vi "client.vi"() -> ()   [LabVIEW 2015]
uses:
  Control/Queue.ctl
panel:
  in  "Operation":bool
  in  "Channel":enum16{"64X4", "128X4"}(ring)=enum."128X4"
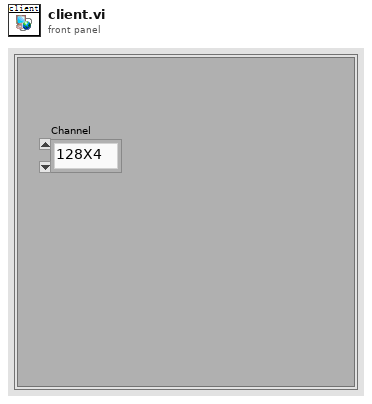
[diagram p1: front panel]
types:
  T1 = typedef "Queue.ctl" = cluster{"Panel":enum16{"None", "Password", "User", "Control", "Monitor", "Operation"}}
  T2 = enum16{"None", "Password", "User", "Control", "Monitor", "Operation"}
  T3 = enum32{"Bad", "Idle", "Run top level", "Running"}
  T4 = typedef "LVRectTypeDef.ctl" = cluster{"Left":i16, "Top":i16, "Right":i16, "Bottom":i16}
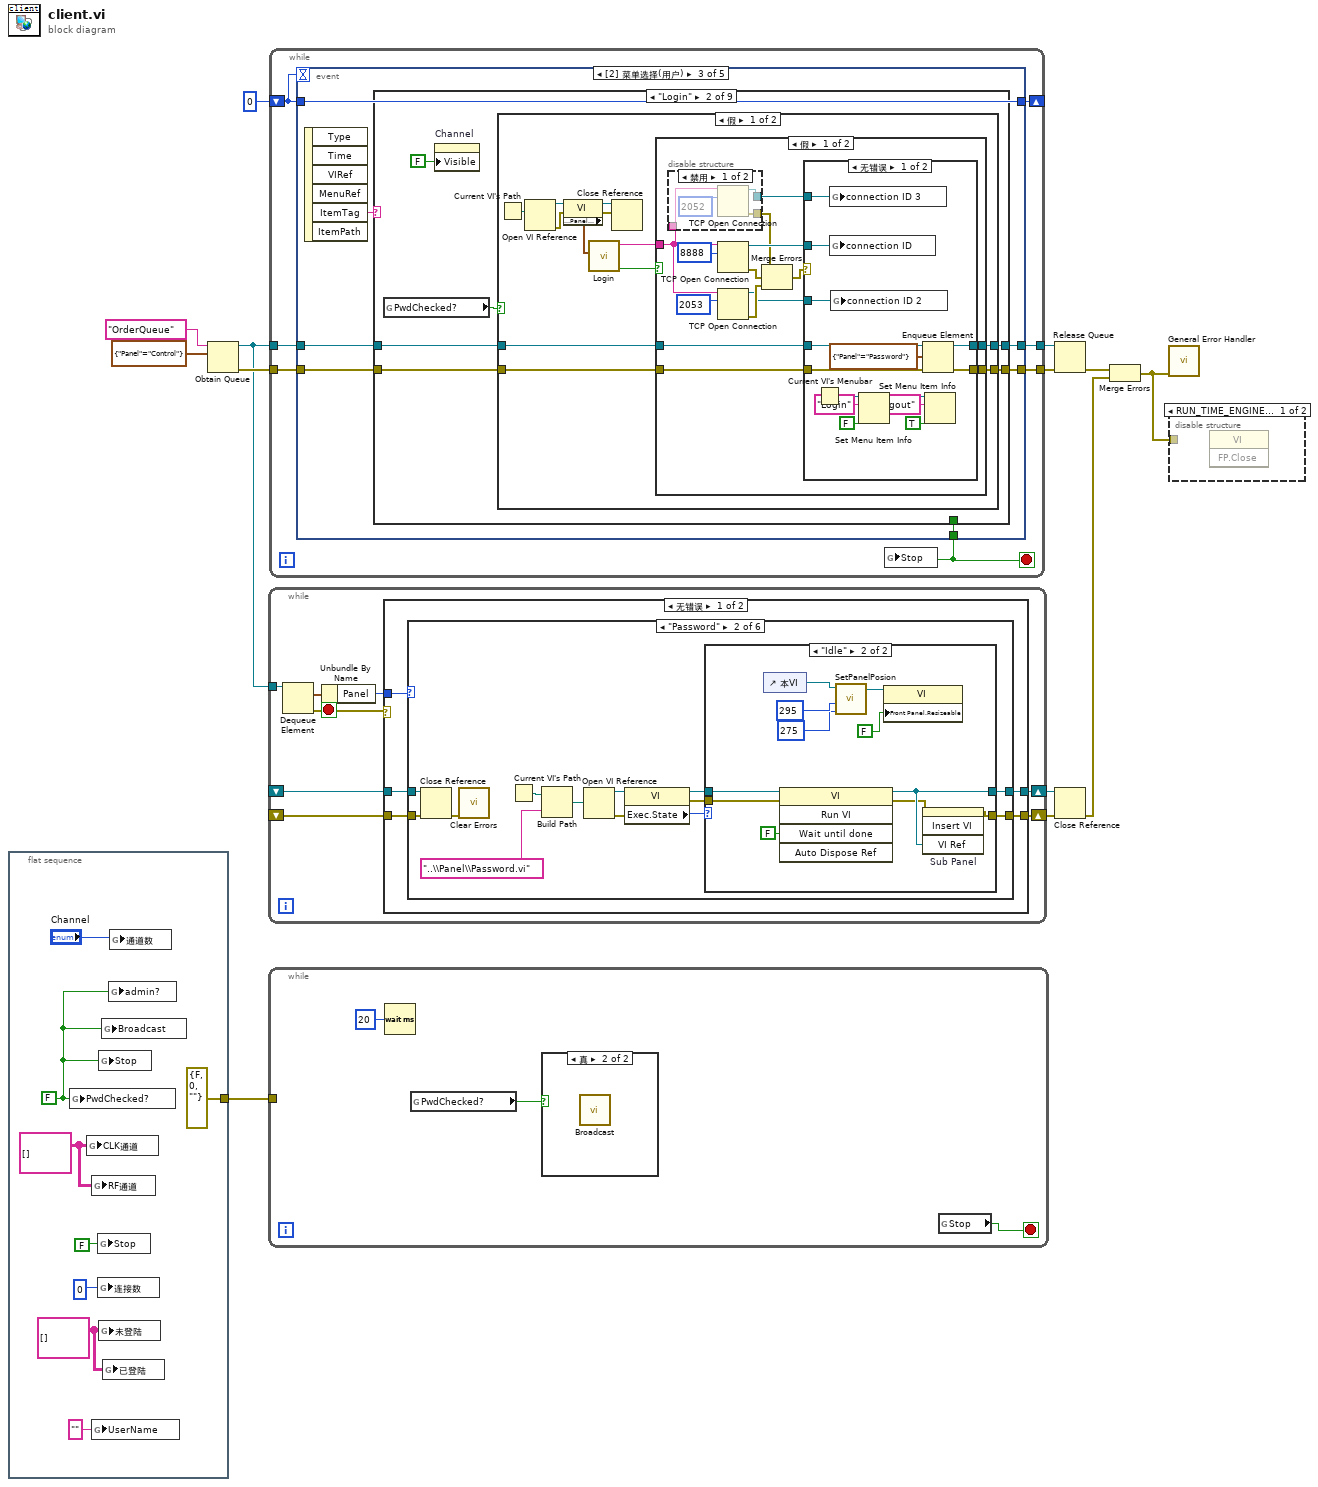
[diagram p0: block diagram]
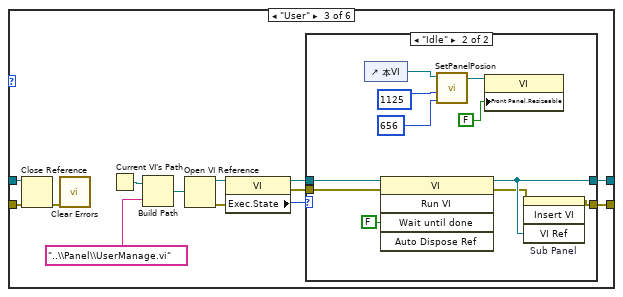
[diagram p6: hidden frame]
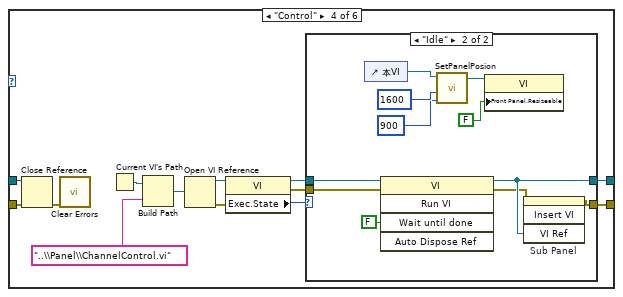
[diagram p8: hidden frame]
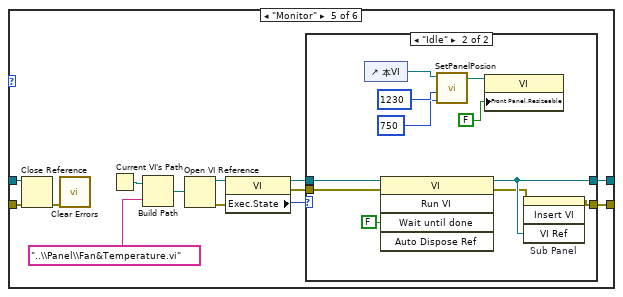
[diagram p10: hidden frame]
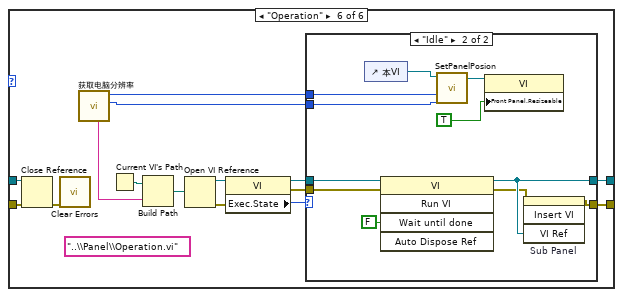
[diagram p12: hidden frame]
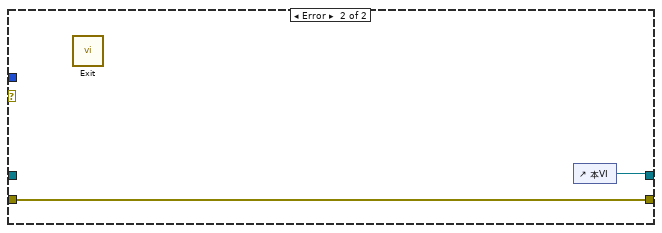
[diagram p14: hidden frame]
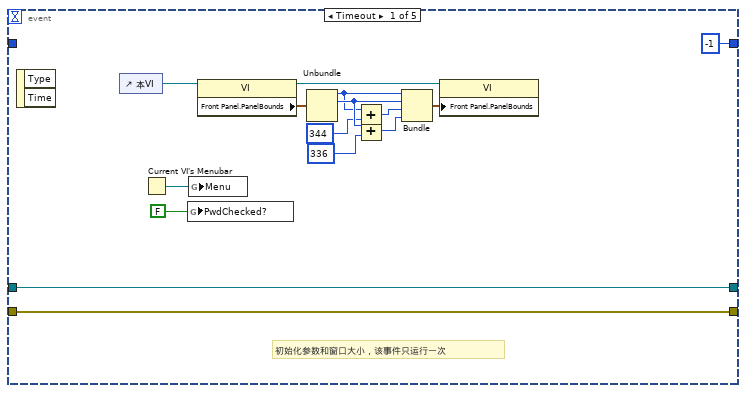
[diagram p15: hidden frame]
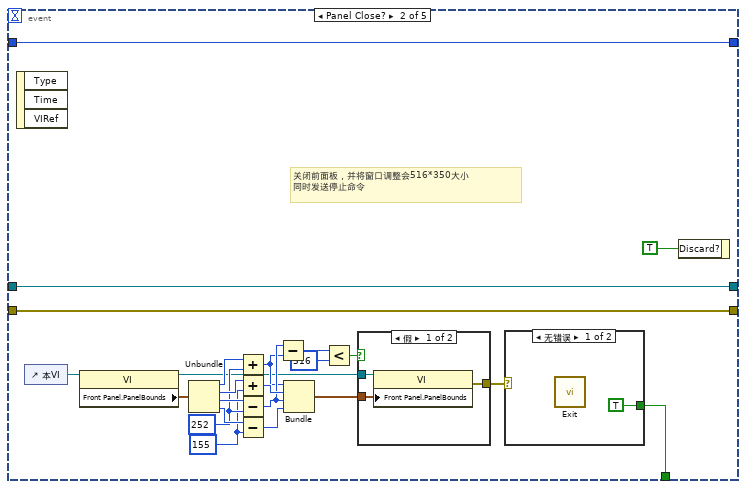
[diagram p16: hidden frame]
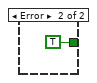
[diagram p18: hidden frame]
diagram:
  n1 = flat-sequence {
    tunnel: [errorcluster {"status"=FALSE, "code"=0, "source"=""} ("error constant")] -> w2
    frame #0 {
      w17 = string[][] [] ("未登陆")
      w20 = string[][] [] ("CLK通道")
      w16 = FALSE ("PwdChecked?")
      n2 = global write "Globalclient.vi" "PwdChecked?"(w16) -> ()
      n3 = global write "Globalclient.vi" "CLK通道"(w20) -> ()
      n4 = global write "Globalclient.vi" "RF通道"(w20) -> ()
      n5 = global write "Globalclient.vi" "UserName"("" ("UserName")) -> ()
      n6 = global write "Globalclient.vi" "Stop"(FALSE ("Stop")) -> ()
      n7 = global write "Globalclient.vi" "连接数"(0 ("连接数")) -> ()
      n8 = global write "Globalclient.vi" "Stop"(w16) -> ()
      n9 = global write "Globalclient.vi" "未登陆"(w17) -> ()
      n10 = global write "Globalclient.vi" "Broadcast"(w16) -> ()
      n11 = global write "Globalclient.vi" "已登陆"(w17) -> ()
      n12 = global write "Globalclient.vi" "admin?"(w16) -> ()
      n13 = global write "Globalclient.vi" "通道数"("Channel") -> ()
    }
  }
  n14 = Obtain Queue(name (unnamed)="OrderQueue" ("名称（未命名）"), element data type=T1 {"Panel"=enum."Control"}) -> (queue out=w8:refnum<queue>, error out=w11:errorcluster)  [unwired: 3 in, 1 out]
  n15 = while {
    tunnel: w8 -> [w29]
    shift-right: [w26] -> w7
    shift-left: _ -> [w24]
    shift-right: [w25] -> w6
    shift-left: _ -> [w23]
    stop <- w22 stop-if-true
    n16 = Dequeue Element(queue=w29) -> (element=w28:T1, error out=w22:errorcluster)  [unwired: 2 in, 2 out]
    n17 = Unbundle By Name(w28) -> ("Panel"=w27:T2)
    n18 = case shown="无错误" w22 {
      tunnel: w27 -> [w30 _]
      tunnel: [w34 w168] -> w26
      tunnel: [w33 w169] -> w25
      tunnel: w24 -> [w32 _]
      tunnel: w23 -> [w31 w169]
      frame No Error {
        n19 = case shown="\"Password\"" w30 {
          tunnel: [_ w47 w73 w99 w125 w154] -> w34
          tunnel: [w35 w45 w71 w97 w123 w152] -> w33
          tunnel: w32 -> [_ w44 w70 w96 w122 w151]
          tunnel: w31 -> [w35 w43 w69 w95 w121 w150]
          frame "None", Default {
          }
          frame "Password" {
            n20 = Close Reference(reference=w44, error in (no error)=w43) -> (error out=w46:errorcluster)
            n21 = call <vilib>:"Clear Errors.vi"("error in (no error)"=w46) -> ()  [unwired: 5 in, 2 out]
            n22 = Current VI's Path() -> (path=w37:path)
            n23 = Build Path(base path=w37, name or relative path="..\\Panel\\Password.vi" ("名称或相对路径")) -> (appended path=w36:path)
            n24 = Open VI Reference(vi path=w36) -> (vi reference=w42:refnum<vi>, error out=w40:errorcluster)  [unwired: 5 in]
            n25 = property class="VI"(reference=w42, error in=w40) -> (reference out=w41:refnum<vi>, error out=w39:errorcluster, "Exec.State"=w38:T3)
            n26 = case shown="\"Idle\"" w38 {
              tunnel: [w49 w60] -> w47
              tunnel: [w50 w59] -> w45
              tunnel: w41 -> [w49 w57]
              tunnel: w39 -> [w50 w56]
              frame "Bad", Default {
              }
              frame "Idle" {
                n27 = control-ref of="本VI"() -> (w55:refnum<vi>)
                n28 = invoke class="VI" method="Run VI"(reference=w57, error in=w56, "Wait until done"=FALSE ("结束前等待")) -> (reference out=w60:refnum<vi>, error out=w58:errorcluster)  [unwired: 2 in, 3 out]
                n29 = call "SetPanelPosion.vi"("Bottom"=i16 275, "Right"=i16 295, "VI ref in"=w55) -> ("VI ref out"=w52:refnum<vi>)  [unwired: 8 in]
                n30 = property class="VI"(reference=w52, "Front Panel.Resizeable"=FALSE ("Front Panel Window:Resizable")) -> ()  [unwired: 1 in, 2 out]
                n31 = invoke on="Sub Panel" class="SubPnl" method="Insert VI"(error in=w58, "VI Ref"=w60) -> (error out=w59:errorcluster)  [unwired: 2 in, 3 out]
              }
            }
          }
          frame "User" {
            n32 = Close Reference(reference=w70, error in (no error)=w69) -> (error out=w72:errorcluster)
            n33 = call <vilib>:"Clear Errors.vi"("error in (no error)"=w72) -> ()  [unwired: 5 in, 2 out]
            n34 = Current VI's Path() -> (path=w63:path)
            n35 = Build Path(base path=w63, name or relative path="..\\Panel\\UserManage.vi" ("名称或相对路径")) -> (appended path=w62:path)
            n36 = Open VI Reference(vi path=w62) -> (vi reference=w68:refnum<vi>, error out=w66:errorcluster)  [unwired: 5 in]
            n37 = property class="VI"(reference=w68, error in=w66) -> (reference out=w67:refnum<vi>, error out=w65:errorcluster, "Exec.State"=w64:T3)
            n38 = case shown="\"Idle\"" w64 {
              tunnel: [w75 w86] -> w73
              tunnel: [w76 w85] -> w71
              tunnel: w67 -> [w75 w83]
              tunnel: w65 -> [w76 w82]
              frame "Bad", Default {
              }
              frame "Idle" {
                n39 = control-ref of="本VI"() -> (w81:refnum<vi>)
                n40 = invoke class="VI" method="Run VI"(reference=w83, error in=w82, "Wait until done"=FALSE ("结束前等待")) -> (reference out=w86:refnum<vi>, error out=w84:errorcluster)  [unwired: 2 in, 3 out]
                n41 = call "SetPanelPosion.vi"("Bottom"=i16 656, "Right"=i16 1125, "VI ref in"=w81) -> ("VI ref out"=w78:refnum<vi>)  [unwired: 8 in]
                n42 = property class="VI"(reference=w78, "Front Panel.Resizeable"=FALSE ("Front Panel Window:Resizable")) -> ()  [unwired: 1 in, 2 out]
                n43 = invoke on="Sub Panel" class="SubPnl" method="Insert VI"(error in=w84, "VI Ref"=w86) -> (error out=w85:errorcluster)  [unwired: 2 in, 3 out]
              }
            }
          }
          frame "Control" {
            n44 = Close Reference(reference=w96, error in (no error)=w95) -> (error out=w98:errorcluster)
            n45 = call <vilib>:"Clear Errors.vi"("error in (no error)"=w98) -> ()  [unwired: 5 in, 2 out]
            n46 = Current VI's Path() -> (path=w89:path)
            n47 = Build Path(base path=w89, name or relative path="..\\Panel\\ChannelControl.vi" ("名称或相对路径")) -> (appended path=w88:path)
            n48 = Open VI Reference(vi path=w88) -> (vi reference=w94:refnum<vi>, error out=w92:errorcluster)  [unwired: 5 in]
            n49 = property class="VI"(reference=w94, error in=w92) -> (reference out=w93:refnum<vi>, error out=w91:errorcluster, "Exec.State"=w90:T3)
            n50 = case shown="\"Idle\"" w90 {
              tunnel: [w101 w112] -> w99
              tunnel: [w102 w111] -> w97
              tunnel: w93 -> [w101 w109]
              tunnel: w91 -> [w102 w108]
              frame "Bad", Default {
              }
              frame "Idle" {
                n51 = control-ref of="本VI"() -> (w107:refnum<vi>)
                n52 = invoke class="VI" method="Run VI"(reference=w109, error in=w108, "Wait until done"=FALSE ("结束前等待")) -> (reference out=w112:refnum<vi>, error out=w110:errorcluster)  [unwired: 2 in, 3 out]
                n53 = call "SetPanelPosion.vi"("Bottom"=i16 900, "Right"=i16 1600, "VI ref in"=w107) -> ("VI ref out"=w104:refnum<vi>)  [unwired: 8 in]
                n54 = property class="VI"(reference=w104, "Front Panel.Resizeable"=FALSE ("Front Panel Window:Resizable")) -> ()  [unwired: 1 in, 2 out]
                n55 = invoke on="Sub Panel" class="SubPnl" method="Insert VI"(error in=w110, "VI Ref"=w112) -> (error out=w111:errorcluster)  [unwired: 2 in, 3 out]
              }
            }
          }
          frame "Monitor" {
            n56 = Close Reference(reference=w122, error in (no error)=w121) -> (error out=w124:errorcluster)
            n57 = call <vilib>:"Clear Errors.vi"("error in (no error)"=w124) -> ()  [unwired: 5 in, 2 out]
            n58 = Current VI's Path() -> (path=w115:path)
            n59 = Build Path(base path=w115, name or relative path="..\\Panel\\Fan&Temperature.vi" ("名称或相对路径")) -> (appended path=w114:path)
            n60 = Open VI Reference(vi path=w114) -> (vi reference=w120:refnum<vi>, error out=w118:errorcluster)  [unwired: 5 in]
            n61 = property class="VI"(reference=w120, error in=w118) -> (reference out=w119:refnum<vi>, error out=w117:errorcluster, "Exec.State"=w116:T3)
            n62 = case shown="\"Idle\"" w116 {
              tunnel: [w127 w138] -> w125
              tunnel: [w128 w137] -> w123
              tunnel: w119 -> [w127 w135]
              tunnel: w117 -> [w128 w134]
              frame "Bad", Default {
              }
              frame "Idle" {
                n63 = control-ref of="本VI"() -> (w133:refnum<vi>)
                n64 = invoke class="VI" method="Run VI"(reference=w135, error in=w134, "Wait until done"=FALSE ("结束前等待")) -> (reference out=w138:refnum<vi>, error out=w136:errorcluster)  [unwired: 2 in, 3 out]
                n65 = call "SetPanelPosion.vi"("Bottom"=i16 750, "Right"=i16 1230, "VI ref in"=w133) -> ("VI ref out"=w130:refnum<vi>)  [unwired: 8 in]
                n66 = property class="VI"(reference=w130, "Front Panel.Resizeable"=FALSE ("Front Panel Window:Resizable")) -> ()  [unwired: 1 in, 2 out]
                n67 = invoke on="Sub Panel" class="SubPnl" method="Insert VI"(error in=w136, "VI Ref"=w138) -> (error out=w137:errorcluster)  [unwired: 2 in, 3 out]
              }
            }
          }
          frame "Operation" {
            (unwired) "..\\Panel\\Operation.vi" ("名称或相对路径")
            n68 = Close Reference(reference=w151, error in (no error)=w150) -> (error out=w153:errorcluster)
            n69 = call <vilib>:"Clear Errors.vi"("error in (no error)"=w153) -> ()  [unwired: 5 in, 2 out]
            n70 = call "获取电脑分辨率.vi"() -> ("宽"=w140:i32, "长"=w141:i32, "子面板路径"=w142:string)  [unwired: 9 in]
            n71 = Current VI's Path() -> (path=w144:path)
            n72 = Build Path(base path=w144, name or relative path=w142) -> (appended path=w143:path)
            n73 = Open VI Reference(vi path=w143) -> (vi reference=w149:refnum<vi>, error out=w147:errorcluster)  [unwired: 5 in]
            n74 = property class="VI"(reference=w149, error in=w147) -> (reference out=w148:refnum<vi>, error out=w146:errorcluster, "Exec.State"=w145:T3)
            n75 = case shown="\"Idle\"" w145 {
              tunnel: [w155 w166] -> w154
              tunnel: [w156 w165] -> w152
              tunnel: w148 -> [w155 w163]
              tunnel: w146 -> [w156 w162]
              tunnel: w141 -> [_ w158]
              tunnel: w140 -> [_ w157]
              frame "Bad", Default {
              }
              frame "Idle" {
                n76 = control-ref of="本VI"() -> (w161:refnum<vi>)
                n77 = invoke class="VI" method="Run VI"(reference=w163, error in=w162, "Wait until done"=FALSE ("结束前等待")) -> (reference out=w166:refnum<vi>, error out=w164:errorcluster)  [unwired: 2 in, 3 out]
                n78 = call "SetPanelPosion.vi"("Bottom"=w157, "Right"=w158, "VI ref in"=w161) -> ("VI ref out"=w160:refnum<vi>)  [unwired: 8 in]
                n79 = property class="VI"(reference=w160, "Front Panel.Resizeable"=TRUE ("Front Panel Window:Resizable")) -> ()  [unwired: 1 in, 2 out]
                n80 = invoke on="Sub Panel" class="SubPnl" method="Insert VI"(error in=w164, "VI Ref"=w166) -> (error out=w165:errorcluster)  [unwired: 2 in, 3 out]
              }
            }
          }
        }
      }
      frame Error {
        n81 = call "Exit.vi"() -> ()  [unwired: 12 in]
        n82 = control-ref of="本VI"() -> (w168:refnum<vi>)
      }
    }
  }
  n83 = while {
    tunnel: w2 -> [_]
    stop <- w170 stop-if-true
    n84 = Wait (ms)(milliseconds to wait=u32 20) -> ()  [unwired: 1 out]
    n85 = global read "Globalclient.vi" "PwdChecked?"() -> (w172:bool)
    n86 = case shown="真" w172 {
      frame False {
      }
      frame True {
        n87 = call "Broadcast.vi"() -> ()  [unwired: 20 in]
      }
    }
    n88 = global read "Globalclient.vi" "Stop"() -> (w170:bool)
  }
  n89 = while {
    tunnel: w8 -> [w179]
    tunnel: [w178] -> w10
    tunnel: w11 -> [w177]
    tunnel: [w176] -> w9
    shift-right: [w175] -> _
    shift-left: 0 -> [w174]
    stop <- w173 stop-if-true
    n90 = event shown="[2] 菜单选择(用户)" {
      selector: _ -> [_ _ _ _ _]
      dyn-events: _ -> [_ _ _ _ _]
      timeout: w174 -> [_ _ _ _ _]
      tunnel: [_ w214 w228 _ _] -> w173
      tunnel: w179 -> [w193 w216 w227 w393 w399]
      tunnel: [w194 w217 w226 w394 w396] -> w178
      tunnel: w177 -> [w194 w217 w225 w394 w397]
      tunnel: [w193 w216 w224 w393 w398] -> w176
      tunnel: [-1 w213 w223 _ _] -> w175
      tunnel: w174 -> [_ w213 w223 _ _]
      event Timeout {
        # "初始化参数和窗口大小，该事件只运行一次"
        n91 = event-data() -> ()  [unwired: 1 in, 2 out]
        n92 = control-ref of="本VI"() -> (w192:refnum<vi>)
        n93 = Current VI's Menubar() -> (w181:refnum<k9>)
        n94 = global write "Globalclient.vi" "PwdChecked?"(FALSE ("PwdChecked?")) -> ()
        n95 = global write "Globalclient.vi" "Menu"(w181) -> ()
        n96 = property class="VI"(reference=w192) -> (reference out=w183:refnum<vi>, "Front Panel.PanelBounds"=w184:T4)  [unwired: 1 in, 1 out]
        n97 = Unbundle(w184) -> ("Left"=w187:i16, "Top"=w188:i16)  [unwired: 2 out]
        n98 = Add(x=w187, y=i16 344 ("Right")) -> (x+y=w189:i16)
        n99 = Add(x=w188, y=i16 336 ("Bottom")) -> (x+y=w190:i16)
        n100 = Bundle("Left"=w187, "Top"=w188, w189, w190) -> (w191:cluster{"Left":i16, "Top":i16, i16, i16})  [unwired: 1 in]
        n101 = property class="VI"(reference=w183, "Front Panel.PanelBounds"=w191) -> ()  [unwired: 1 in, 2 out]
      }
      event Panel Close? {
        w202 = i16 155 ("Bottom")
        w203 = i16 252 ("Right")
        # "关闭前面板，并将窗口调整会516*350大小\n同时发送停止命令"
        n102 = event-data() -> ()  [unwired: 1 in, 3 out]
        n103 = control-ref of="本VI"() -> (w211:refnum<vi>)
        n104 = property class="VI"(reference=w211) -> (reference out=w197:refnum<vi>, "Front Panel.PanelBounds"=w208:T4)  [unwired: 1 in, 1 out]
        n105 = Unbundle(w208) -> ("Left"=w209:i16, "Top"=w206:i16, "Right"=w205:i16, "Bottom"=w204:i16)
        n106 = Add(x=w209, y=w203) -> (x+y=w199:i16)
        n107 = Add(x=w206, y=w202) -> (x+y=w207:i16)
        n108 = Subtract(x=w205, y=w203) -> (x-y=w200:i16)
        n109 = Subtract(x=w204, y=w202) -> (x-y=w210:i16)
        n110 = Subtract(x=w200, y=w199) -> (x-y=w201:i16)
        n111 = Bundle(w199, w207, w200, w210) -> (w196:cluster{i16, i16, i16, i16})  [unwired: 1 in]
        n112 = Less?(x=w201, y=i16 516) -> (x < y?=w195:bool)
        n113 = case shown="假" w195 {
          tunnel: w197 -> [w220 _]
          tunnel: w196 -> [w219 _]
          tunnel: [w218 _] -> w212
          frame False {
            n114 = property class="VI"(reference=w220, "Front Panel.PanelBounds"=w219) -> (error out=w218:errorcluster)  [unwired: 1 in, 1 out]
          }
          frame True {
          }
        }
        n115 = case shown="无错误" w212 {
          tunnel: [TRUE TRUE] -> w214
          frame No Error {
            n116 = call "Exit.vi"() -> ()  [unwired: 12 in]
          }
          frame Error {
          }
        }
        n117 = event-data("Discard?"=TRUE ("放弃？")) -> ()  [unwired: 1 in, 1 out]
      }
      event Menu Selection (User) {
        n118 = event-data() -> ("ItemTag"=w229:string)  [unwired: 1 in, 5 out]
        n119 = case shown="\"Login\"" w229 {
          tunnel: [_ _ _ _ _ _ _ w376 _] -> w228
          tunnel: w227 -> [w231 w237 w293 w335 w340 w345 w349 w378 w390]
          tunnel: [w230 w236 w291 w332 w337 w342 w346 w377 w391] -> w226
          tunnel: w225 -> [w230 w235 w292 w333 w338 w343 w347 w377 w391]
          tunnel: [w231 w234 w290 w334 w339 w344 w348 w378 w390] -> w224
          frame "假", Default {
          }
          frame "Login" {
            n120 = global read "Globalclient.vi" "PwdChecked?"() -> (w233:bool)
            n121 = property on="Channel" class="Enum (严格)"("Visible"=FALSE ("可见")) -> ()  [unwired: 2 in, 2 out]
            n122 = case shown="假" w233 {
              tunnel: w237 -> [w244 w289]
              tunnel: [w243 w288] -> w236
              tunnel: w235 -> [w242 w288]
              tunnel: [w241 w289] -> w234
              frame False {
                n123 = Current VI's Path() -> (path=w249:path)
                n124 = Open VI Reference(vi path=w249) -> (vi reference=w248:refnum<vi>, error out=w247:errorcluster)  [unwired: 5 in]
                n125 = property class="VI"(reference=w248, error in=w247) -> (reference out=w245:refnum<vi>, error out=w246:errorcluster, "Front Panel.PanelBounds"=w240:T4)
                n126 = call "Login.vi"("窗口边界"=w240) -> ("drop?"=w238:bool, "User IP"=w239:string)  [unwired: 9 in]
                n127 = Close Reference(reference=w245, error in (no error)=w246) -> ()  [unwired: 1 out]
                n128 = case shown="假" w238 {
                  tunnel: w239 -> [w252 _]
                  tunnel: w244 -> [w261 w286]
                  tunnel: [w260 w285] -> w243
                  tunnel: w242 -> [w259 w285]
                  tunnel: [w258 w286] -> w241
                  frame False {
                    n129 = disable-structure shown="禁用" {
                      disable-tunnel: [w266 _] -> w253
                      disable-tunnel: w252 -> [w265 _]
                      disable-tunnel: [w264 _] -> w251
                      frame Disabled {
                        n130 = TCP Open Connection(address=w265, remote port or service name=u32 2052 ("远程端口或服务名称")) -> (connection ID=w266:refnum<k5>, error out=w264:errorcluster)  [unwired: 3 in]
                      }
                      frame Enabled {
                      }
                    }
                    n131 = TCP Open Connection(address=w252, remote port or service name=u32 8888 ("远程端口或服务名称")) -> (connection ID=w262:refnum<k5>, error out=w257:errorcluster)  [unwired: 3 in]
                    n132 = TCP Open Connection(address=w252, remote port or service name=u32 2053 ("远程端口或服务名称")) -> (connection ID=w254:refnum<k5>, error out=w256:errorcluster)  [unwired: 3 in]
                    n133 = Merge Errors(w251, w257, w256) -> (w255:errorcluster)
                    n134 = case shown="无错误" w255 {
                      tunnel: w262 -> [w271 _]
                      tunnel: w261 -> [w281 w284]
                      tunnel: [w279 w283] -> w260
                      tunnel: w259 -> [w280 w283]
                      tunnel: [w278 w284] -> w258
                      tunnel: w254 -> [w269 _]
                      tunnel: w253 -> [w268 _]
                      frame No Error {
                        n135 = Current VI's Menubar() -> (w277:refnum<k9>)
                        n136 = global write "Globalclient.vi" "connection ID 3"(w268) -> ()
                        n137 = global write "Globalclient.vi" "connection ID"(w271) -> ()
                        n138 = global write "Globalclient.vi" "connection ID 2"(w269) -> ()
                        n139 = Set Menu Item Info(7:"Login" ("项名称"), 9:FALSE ("已启用"), 11:w277) -> (3:w276:refnum<k9>)  [unwired: 4 in, 1 out]
                        n140 = Enqueue Element(queue=w281, element=T1 {"Panel"=enum."Password"}, error in (no error)=w280) -> (queue out=w278:refnum<queue>, error out=w279:errorcluster)  [unwired: 1 in, 1 out]
                        n141 = Set Menu Item Info(7:"Logout" ("项名称"), 9:TRUE ("已启用"), 11:w276) -> ()  [unwired: 4 in, 2 out]
                      }
                      frame Error {
                        n142 = One Button Dialog(message="Link failure!" ("消息")) -> ()  [unwired: 1 in, 1 out]
                      }
                    }
                  }
                  frame True {
                  }
                }
              }
              frame True {
                n143 = One Button Dialog(message="Server connected!" ("消息")) -> ()  [unwired: 1 in, 1 out]
              }
            }
          }
          frame "Logout" {
            w300 = i16 155 ("Bottom")
            w301 = i16 252 ("Right")
            n144 = control-ref of="本VI"() -> (w311:refnum<vi>)
            n145 = property class="VI"(reference=w311) -> (reference out=w307:refnum<vi>, "Front Panel.PanelBounds"=w308:T4)  [unwired: 1 in, 1 out]
            n146 = Unbundle(w308) -> ("Left"=w309:i16, "Top"=w304:i16, "Right"=w303:i16, "Bottom"=w302:i16)
            n147 = Add(x=w309, y=w301) -> (x+y=w295:i16)
            n148 = Add(x=w304, y=w300) -> (x+y=w305:i16)
            n149 = Subtract(x=w303, y=w301) -> (x-y=w296:i16)
            n150 = Subtract(x=w302, y=w300) -> (x-y=w310:i16)
            n151 = Subtract(x=w296, y=w295) -> (x-y=w297:i16)
            n152 = Bundle(w295, w305, w296, w310) -> (w306:cluster{i16, i16, i16, i16})  [unwired: 1 in]
            n153 = Less?(x=w297, y=i16 516) -> (x < y?=w299:bool)
            n154 = case shown="真" w299 {
              tunnel: w307 -> [w314 _]
              tunnel: w306 -> [w313 _]
              tunnel: [w312 _] -> w298
              frame False {
                n155 = property class="VI"(reference=w314, "Front Panel.PanelBounds"=w313) -> (error out=w312:errorcluster)  [unwired: 1 in, 1 out]
              }
              frame True {
              }
            }
            n156 = case shown="无错误" w298 {
              tunnel: w293 -> [w318 w330]
              tunnel: w292 -> [w317 w329]
              tunnel: [w317 w329] -> w291
              tunnel: [w318 w330] -> w290
              frame No Error {
                n157 = global write "Globalclient.vi" "PwdChecked?"(FALSE ("PwdChecked?")) -> ()
                n158 = invoke on="Sub Panel" class="SubPanel" method="Remove VI"() -> ()  [unwired: 3 in, 3 out]
                n159 = Current VI's Menubar() -> (w327:refnum<k9>)
                n160 = call "Exit.vi"() -> ()  [unwired: 12 in]
                n161 = Set Menu Item Info(7:"Login" ("项名称"), 9:TRUE ("已启用"), 11:w327) -> (0:w322:errorcluster, 3:w326:refnum<k9>)  [unwired: 4 in]
                n162 = Set Menu Item Info(7:"Logout" ("项名称"), 8:w322, 9:FALSE ("已启用"), 11:w326) -> (0:w321:errorcluster, 3:w323:refnum<k9>)  [unwired: 3 in]
                n163 = Delete Menu Items(6:w321, 7:"Operation" ("项"), 9:w323) -> (0:w315:errorcluster)  [unwired: 1 in, 1 out]
                n164 = call <vilib>:"Clear Errors.vi"("error in (no error)"=w315) -> ()  [unwired: 5 in, 2 out]
              }
              frame Error {
              }
            }
          }
          frame "User" {
            n165 = Enqueue Element(queue=w335, element=T1 {"Panel"=enum."User"}, error in (no error)=w333) -> (queue out=w334:refnum<queue>, error out=w332:errorcluster)  [unwired: 1 in, 1 out]
          }
          frame "Control" {
            n166 = Enqueue Element(queue=w340, element=T1 {"Panel"=enum."Control"}, error in (no error)=w338) -> (queue out=w339:refnum<queue>, error out=w337:errorcluster)  [unwired: 1 in, 1 out]
          }
          frame "Monitor" {
            n167 = Enqueue Element(queue=w345, element=T1 {"Panel"=enum."Monitor"}, error in (no error)=w343) -> (queue out=w344:refnum<queue>, error out=w342:errorcluster)  [unwired: 1 in, 1 out]
          }
          frame "Operation" {
            n168 = disable-structure shown="Enabled" {
              disable-tunnel: w349 -> [w353 w356]
              disable-tunnel: [w352 w356] -> w348
              disable-tunnel: w347 -> [w351 w355]
              disable-tunnel: [w350 w355] -> w346
              frame Enabled {
                n169 = Enqueue Element(queue=w353, element=T1 {"Panel"=enum."Operation"}, error in (no error)=w351) -> (queue out=w352:refnum<queue>, error out=w350:errorcluster)  [unwired: 1 in, 1 out]
              }
              frame Disabled {
              }
            }
          }
          frame "Exit" {
            w364 = i16 155 ("Bottom")
            w365 = i16 252 ("Right")
            n170 = control-ref of="本VI"() -> (w375:refnum<vi>)
            n171 = property class="VI"(reference=w375) -> (reference out=w371:refnum<vi>, "Front Panel.PanelBounds"=w372:T4)  [unwired: 1 in, 1 out]
            n172 = property on="Channel" class="Enum (严格)"("Visible"=TRUE ("可见")) -> ()  [unwired: 2 in, 2 out]
            n173 = Unbundle(w372) -> ("Left"=w373:i16, "Top"=w368:i16, "Right"=w367:i16, "Bottom"=w366:i16)
            n174 = Add(x=w373, y=w365) -> (x+y=w359:i16)
            n175 = Add(x=w368, y=w364) -> (x+y=w369:i16)
            n176 = Subtract(x=w367, y=w365) -> (x-y=w360:i16)
            n177 = Subtract(x=w366, y=w364) -> (x-y=w374:i16)
            n178 = Subtract(x=w360, y=w359) -> (x-y=w361:i16)
            n179 = Bundle(w359, w369, w360, w374) -> (w370:cluster{i16, i16, i16, i16})  [unwired: 1 in]
            n180 = Less?(x=w361, y=i16 516) -> (x < y?=w363:bool)
            n181 = case shown="真" w363 {
              tunnel: w371 -> [w381 _]
              tunnel: w370 -> [w380 _]
              tunnel: [w379 _] -> w362
              frame False {
                n182 = property class="VI"(reference=w381, "Front Panel.PanelBounds"=w380) -> (error out=w379:errorcluster)  [unwired: 1 in, 1 out]
              }
              frame True {
              }
            }
            n183 = case shown="无错误" w362 {
              tunnel: [TRUE TRUE] -> w376
              frame No Error {
                n184 = call "Exit.vi"() -> ()  [unwired: 12 in]
              }
              frame Error {
              }
            }
          }
          frame "About" {
            n185 = Current VI's Path() -> (path=w389:path)
            n186 = Open VI Reference(vi path=w389) -> (vi reference=w388:refnum<vi>, error out=w387:errorcluster)  [unwired: 5 in]
            n187 = property class="VI"(reference=w388, error in=w387) -> (reference out=w385:refnum<vi>, error out=w386:errorcluster, "Front Panel.PanelBounds"=w384:T4)
            n188 = call "About.vi"("窗口边界"=w384) -> ()  [unwired: 11 in]
            n189 = Close Reference(reference=w385, error in (no error)=w386) -> ()  [unwired: 1 out]
          }
        }
      }
      event "Channel": Value Change {
        n190 = event-data() -> ("NewVal"=w392:enum16{"64X4", "128X4"})  [unwired: 1 in, 5 out]
        n191 = global write "Globalclient.vi" "通道数"(w392) -> ()
      }
      event "Operation": Value Change {
        n192 = event-data() -> ()  [unwired: 1 in, 6 out]
        n193 = Enqueue Element(queue=w399, element=T1 {"Panel"=enum."Operation"}, error in (no error)=w397) -> (queue out=w398:refnum<queue>, error out=w396:errorcluster)  [unwired: 1 in, 1 out]
      }
    }
    n194 = global write "Globalclient.vi" "Stop"(w173) -> ()
  }
  n195 = Release Queue(queue=w9, error in (no error)=w10) -> (error out=w5:errorcluster)  [unwired: 1 in, 2 out]
  n196 = Close Reference(reference=w7, error in (no error)=w6) -> (error out=w4:errorcluster)
  n197 = Merge Errors(w5, w4) -> (w1:errorcluster)
  n198 = call <vilib>:"General Error Handler.vi"("error in (no error)"=w1) -> ()  [unwired: 10 in, 5 out]
  n199 = disable-structure shown="RUN_TIME_ENGINE==True" {
    disable-tunnel: w1 -> [_ _]
    frame condition #0 {
      n200 = invoke class="VI" method="FP.Close"() -> ()  [unwired: 3 in, 3 out]
    }
    frame condition #1 (active) {
    }
  }
